vi "Pre Launch Init.vi"(11 "GRAFICAR_SEÑAL_ACTUALIZABLE in":refnum<class "GRAFICAR_SEÑAL_ACTUALIZABLE.lvclass">) -> (0 "error out":errorcluster, 3 "GRAFICAR_SEÑAL_ACTUALIZABLE out":refnum<class "GRAFICAR_SEÑAL_ACTUALIZABLE.lvclass">)   [LabVIEW 2019, in "GRAFICAR_SEÑAL_ACTUALIZABLE.lvlib" / "GRAFICAR_SEÑAL_ACTUALIZABLE.lvclass"]
doc: "(<B>Filename</B>: Actor Framework.lvlib:Actor.lvclass:Pre Launch Init.vi)\n\nDefines behavior that occurs after the Launch Nested Actor method is invoked but before the actor's Actor Core method begins running.\n\nBy default, this method does nothing. A descendant class may override it to define behavior."
uses:
  <vilib>/ActorFramework/Actor/Actor.lvclass
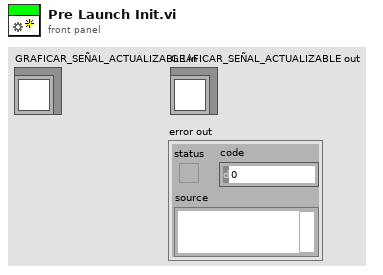
[diagram p1: front panel]
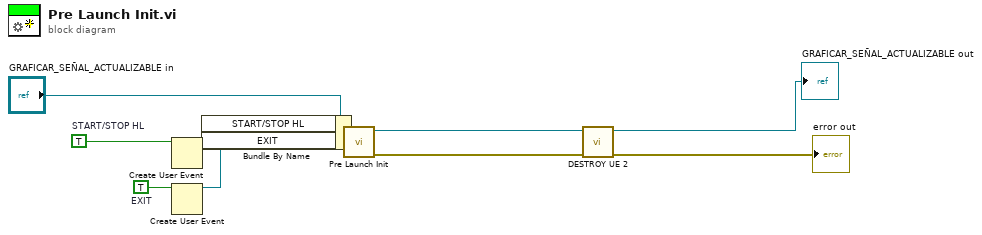
[diagram p0: block diagram]
diagram:
  w8 = TRUE  # EXIT
  w9 = TRUE  # START/STOP HL
  n1 = Create User Event(user event datatype=w9) -> (user event=w6:refnum<user-event>)  [unwired: 1 in, 1 out]
  n2 = Create User Event(user event datatype=w8) -> (user event=w5:refnum<user-event>)  [unwired: 1 in, 1 out]
  n3 = Bundle By Name(cluster="GRAFICAR_SEÑAL_ACTUALIZABLE in", "START/STOP HL"=w6, "EXIT"=w5) -> (w7:refnum<class "GRAFICAR_SEÑAL_ACTUALIZABLE.lvclass">)
  n4 = call-parent "Pre Launch Init.vi"("Actor in"=w7) -> ("error out"=w3:errorcluster, "Actor out"=w4:refnum<class "GRAFICAR_SEÑAL_ACTUALIZABLE.lvclass">)  [unwired: 9 in]
  n5 = call "DESTROY UE 2.vi"("error in (no error)"=w3, "GRAFICAR_SEÑAL_ACTUALIZABLE in"=w4) -> ("error out"=→"error out":errorcluster, "GRAFICAR_SEÑAL_ACTUALIZABLE out"=→"GRAFICAR_SEÑAL_ACTUALIZABLE out":refnum<class "GRAFICAR_SEÑAL_ACTUALIZABLE.lvclass">)  [unwired: 8 in]
